vi "FTW-TransferClient-Construct.vi"(0 "Username":string, 5 "Password":string, 7 "Remote URI":string, 11 "error in":errorcluster, 12 "Headers":T1[](array[typedef])) -> (4 "Transfer Client":refnum<class "FTW-TransferClient-dotNET.lvclass">, 15 "error out":errorcluster)   [LabVIEW 2013, in "FTW-TransferClient-dotNET.lvclass"]
uses:
  FTW-TransferClient-dotNET.lvclass
  Core/src/Collection/FTW-Collection-KeyValuePair.ctl
  FTW-TransferClient-dotNET.lvclass/FTW-TransferClient-dotNET.ctl
panel:
  # "Inputs"
  # "Outputs"
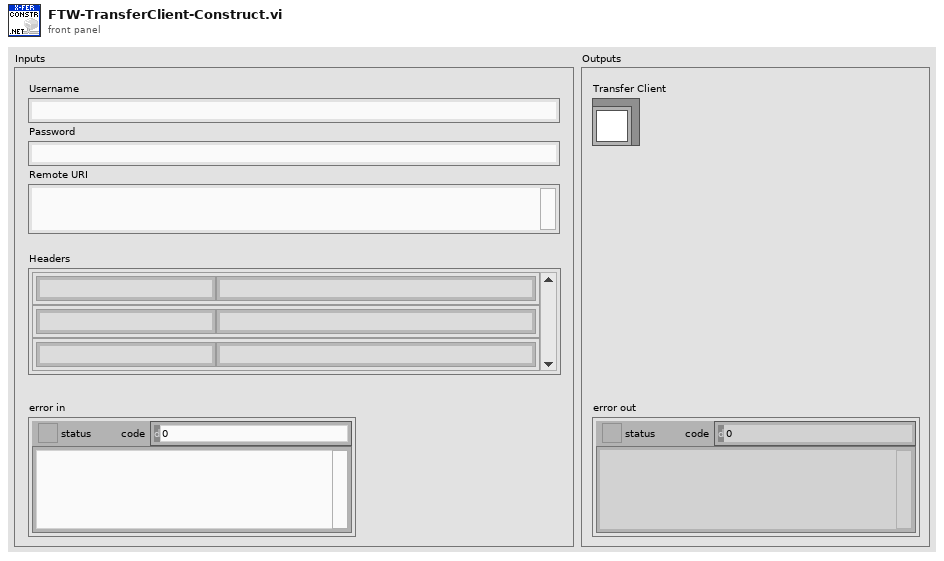
[diagram p1: front panel]
types:
  T1 = typedef "FTW-Collection-KeyValuePair.ctl" = cluster{"Key":string, "Value":string}
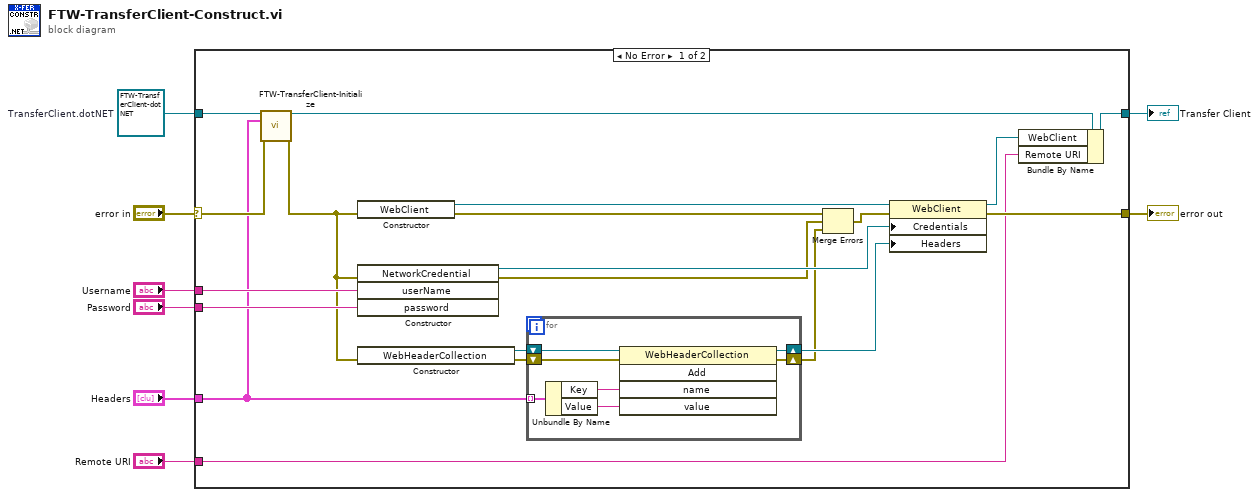
[diagram p0: block diagram]
diagram:
  w5 = refnum<class "FTW-TransferClient-dotNET.lvclass"> refnum  # TransferClient.dotNET
  n1 = case shown="No Error" "error in" {
    selector: "error in" -> [w16 w36]
    tunnel: [w13 w36] -> w7
    tunnel: [w14 w37] -> w6
    tunnel: w5 -> [w17 w37]
    tunnel: "Username" -> [w19 _]
    tunnel: "Password" -> [w18 _]
    tunnel: "Remote URI" -> [w12 _]
    tunnel: "Headers" -> [w9 _]
    frame No Error {
      n2 = call-dynamic "FTW-TransferClient-Initialize.vi"("Transfer Client"=w17, "Headers"=w9, "error in"=w16) -> ("Transfer Client out"=w15:refnum<class "FTW-TransferClient-dotNET.lvclass">, "error out"=w11:errorcluster)  [unwired: 11 in]
      n3 = constructor class="WebClient"(error in=w11) -> (reference out=w28:refnum<k24>, error out=w10:errorcluster)  [unwired: 2 in, 1 out]
      n4 = constructor class="NetworkCredential"(error in=w11, "userName"=w19, "password"=w18) -> (reference out=w27:refnum<k24>, error out=w22:errorcluster)  [unwired: 2 in, 3 out]
      n5 = constructor class="WebHeaderCollection"(error in=w11) -> (reference out=w25:refnum<k24>, error out=w24:errorcluster)  [unwired: 2 in, 1 out]
      n6 = for {
        shift-right: [w33] -> w23
        shift-left: w25 -> [w35]
        shift-right: [w32] -> w21
        shift-left: w24 -> [w34]
        tunnel: w9 -> [w31] mode=indexing
        n7 = Unbundle By Name(w31) -> ("Key"=w30:string, "Value"=w29:string)
        n8 = invoke class="WebHeaderCollection" method="Add"(reference=w35, error in=w34, "name"=w30, "value"=w29) -> (reference out=w33:refnum<k24>, error out=w32:errorcluster)  [unwired: 1 in, 3 out]
      }
      n9 = Merge Errors(w10, w22, w21) -> (w20:errorcluster)
      n10 = property class="WebClient"(reference=w28, error in=w20, "Credentials"=w27, "Headers"=w23) -> (reference out=w26:refnum<k24>, error out=w13:errorcluster)
      n11 = Bundle By Name(cluster=w15, "WebClient"=w26, "Remote URI"=w12) -> (w14:refnum<class "FTW-TransferClient-dotNET.lvclass">)
    }
    frame Error {
    }
  }
  "error out" <- w7
  "Transfer Client" <- w6
